vi "6-CleanFP.vi"   [LabVIEW 2014, in "TestVIs.lvlib"]
uses:
  TestVIs.lvlib
types:
  T1 = enum32{"Top Edges", "Vertical Centers", "Bottom Edges", "Vertical Gap", "Vertical Compress", "Left Edges", "Horizontal Centers", "Right Edges", "Horizontal Gap", "Horizontal Compress"}
  T2 = enum32{"Top Edges", "Vertical Centers", "Bottom Edges", "Left Edges", "Horizontal Centers", "Right Edges"}
  T3 = typedef "LVRectTypeDef.ctl" = cluster{"Left":i16, "Top":i16, "Right":i16, "Bottom":i16}
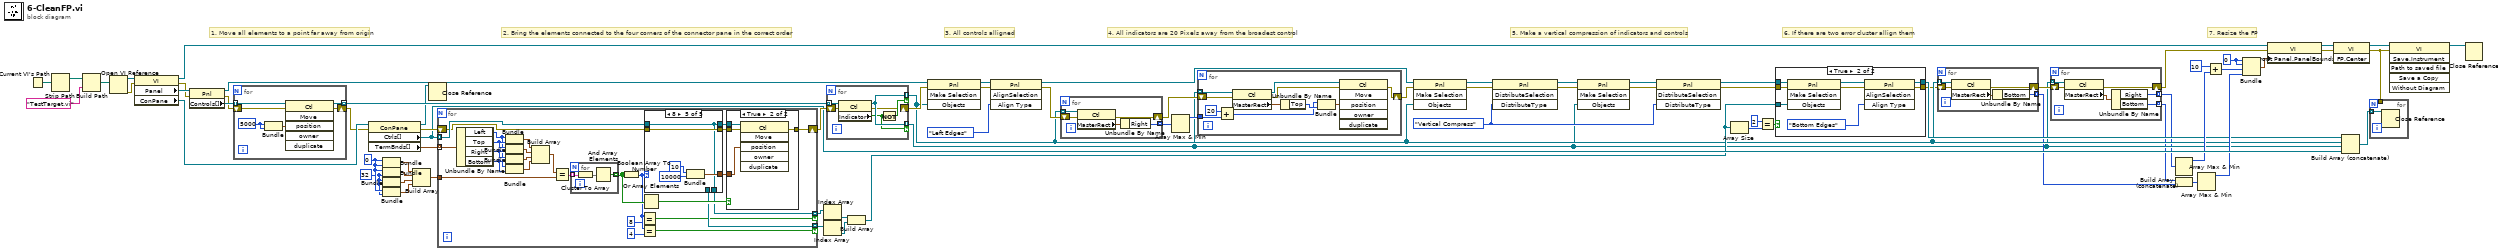
[diagram p0: block diagram]
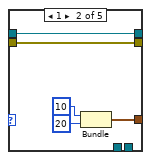
[diagram p4: hidden frame]
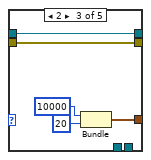
[diagram p5: hidden frame]
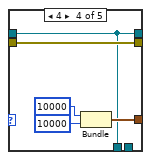
[diagram p6: hidden frame]
diagram:
  w19 = i16 0 ("x")
  w41 = i16 32
  w42 = i16 0
  w50 = T1."Vertical Compress" ("DistributeType")
  # "7. Resize the FP"
  # "6. If there are two error cluster allign them"
  # "2. Bring the elements connected to the four corners of the connector pane in the correct order"
  # "1. Move all elements to a point far away from origin"
  # "5. Make a vertical compression of indicators and controls"
  # "4. All indicators are 20 Pixels away from the broadest control"
  # "3. All controls alligned"
  n1 = Current VI's Path() -> (path=w72:path)
  n2 = Strip Path(path=w72) -> (stripped path=w75:path)  [unwired: 1 out]
  n3 = Build Path(base path=w75, name or relative path="TestTarget.vi") -> (appended path=w73:path)
  n4 = Open VI Reference(vi path=w73) -> (vi reference=w76:refnum<vi>, error out=w49:errorcluster)  [unwired: 5 in]
  n5 = property class="VI"(reference=w76, error in=w49) -> (reference out=w20:refnum<vi>, error out=w70:errorcluster, "Panel"=w71:refnum<vi>, "ConPane"=w45:refnum<vi>)
  n6 = property class="Pnl"(reference=w71, error in=w70) -> (reference out=w69:refnum<vi>, error out=w47:errorcluster, "Controls[]"=w48:refnum<vi>[])
  n7 = for {
    tunnel: w48 -> [w82] mode=indexing
    shift-right: [w80] -> w35
    shift-left: w47 -> [w81]
    tunnel: [w79] -> w46 mode=indexing
    w77 = i16 5000 ("x")
    n8 = Bundle("x"=w77, "x"=w77) -> (w78:cluster{"x":i16, "x":i16})  [unwired: 1 in]
    n9 = invoke class="Ctl" method="Move"(reference=w82, error in=w81, "position"=w78) -> (reference out=w79:refnum<vi>, error out=w80:errorcluster)  [unwired: 3 in, 4 out]
  }
  n10 = property class="ConPane"(reference=w45, error in=w35) -> (reference out=w34:refnum<vi>, error out=w43:errorcluster, "Ctrls[]"=w30:refnum<vi>[], "TermBnds[]"=w44:T3[])
  n11 = Bundle(w42, w42) -> (w40:cluster{i16, i16})  [unwired: 1 in]
  n12 = Bundle(w42, w41) -> (w39:cluster{i16, i16})  [unwired: 1 in]
  n13 = Bundle(w41, w41) -> (w38:cluster{i16, i16})  [unwired: 1 in]
  n14 = Bundle(w42, w41) -> (w37:cluster{i16, i16})  [unwired: 1 in]
  n15 = Build Array(w40, w39, w38, w37) -> (w36:cluster{i16, i16}[])
  n16 = Close Reference(reference=w34) -> ()  [unwired: 1 in, 1 out]
  n17 = for {
    tunnel: w44 -> [w109] mode=indexing
    tunnel: w30 -> [w92] mode=indexing
    tunnel: w36 -> [w99]
    shift-right: [w96] -> w33
    shift-left: w43 -> [w90]
    tunnel: [w89] -> w29 mode=indexing if=w84
    tunnel: [w88] -> w28 mode=indexing if=w83
    n18 = Unbundle By Name(w109) -> ("Left"=w106:i16, "Top"=w108:i16, "Right"=w107:i16, "Bottom"=w105:i16)
    n19 = Bundle("Left"=w106, "Top"=w108) -> (w101:cluster{"Left":i16, "Top":i16})  [unwired: 1 in]
    n20 = Bundle("Top"=w108, "Right"=w107) -> (w102:cluster{"Top":i16, "Right":i16})  [unwired: 1 in]
    n21 = Bundle("Right"=w107, "Bottom"=w105) -> (w103:cluster{"Right":i16, "Bottom":i16})  [unwired: 1 in]
    n22 = Bundle("Left"=w106, "Bottom"=w105) -> (w104:cluster{"Left":i16, "Bottom":i16})  [unwired: 1 in]
    n23 = Build Array(w101, w102, w103, w104) -> (w100:cluster{"Left":i16, "Bottom":i16}[])
    n24 = Equal?(x=w100, y=w99) -> (x = y?=w98:cluster{bool, bool}[])
    n25 = for {
      tunnel: w98 -> [w139] mode=indexing
      tunnel: [w137] -> w95 mode=indexing
      n26 = Cluster To Array(cluster=w139) -> (array=w138:bool[])
      n27 = And Array Elements(Boolean array=w138) -> (logical AND=w137:bool)
    }
    n28 = Boolean Array To Number(Boolean array=w95) -> (number=w87:u32)
    n29 = Equal?(x=w87, y=u32 8) -> (x = y?=w84:bool)
    n30 = Equal?(x=w87, y=u32 4) -> (x = y?=w83:bool)
    n31 = Or Array Elements(Boolean array=w95) -> (logical OR=w97:bool)
    n32 = case shown="8" w87 {
      tunnel: [_ w114 w119 w124 w129] -> w94
      tunnel: [w110 w113 w118 w122 w127] -> w93
      tunnel: w92 -> [w110 w113 w118 w122 w127]
      tunnel: [w111 w112 w117 w123 w128] -> w91
      tunnel: w90 -> [w111 w112 w117 w123 w128]
      tunnel: [_ _ _ _ w127] -> w89
      tunnel: [_ _ _ w122 _] -> w88
      frame 0, Default {
      }
      frame 1 {
        n33 = Bundle("x"=i16 10, "x"=i16 20) -> (w114:cluster{"x":i16, "x":i16})  [unwired: 1 in]
      }
      frame 2 {
        n34 = Bundle("x"=i16 10000, "x"=i16 20) -> (w119:cluster{"x":i16, "x":i16})  [unwired: 1 in]
      }
      frame 4 {
        n35 = Bundle("x"=i16 10000, "x"=i16 10000) -> (w124:cluster{"x":i16, "x":i16})  [unwired: 1 in]
      }
      frame 8 {
        n36 = Bundle("x"=i16 10, "x"=i16 10000) -> (w129:cluster{"x":i16, "x":i16})  [unwired: 1 in]
      }
    }
    n37 = case shown="True" w97 {
      tunnel: w93 -> [_ w136]
      tunnel: w91 -> [w132 w135]
      tunnel: [w132 w134] -> w96
      tunnel: w94 -> [_ w133]
      frame False {
      }
      frame True {
        n38 = invoke class="Ctl" method="Move"(reference=w136, error in=w135, "position"=w133) -> (error out=w134:errorcluster)  [unwired: 3 in, 5 out]
      }
    }
  }
  n39 = Index Array(array=w29) -> (element=w27:refnum<vi>)  [unwired: 1 in]
  n40 = Index Array(array=w28) -> (element=w26:refnum<vi>)  [unwired: 1 in]
  n41 = for {
    tunnel: w46 -> [w145] mode=indexing
    tunnel: [w144] -> w14 mode=indexing if=w143
    tunnel: [w144] -> w10 mode=indexing if=w142
    shift-right: [w140] -> w66
    shift-left: w33 -> [w141]
    n42 = property class="Ctl"(reference=w145, error in=w141) -> (reference out=w144:refnum<vi>, error out=w140:errorcluster, "Indicator"=w142:bool)
    n43 = Not(x=w142) -> (.not. x?=w143:bool)
  }
  n44 = Build Array(w27, w26) -> (w22:refnum<vi>[])
  n45 = invoke class="Pnl" method="Make Selection"(reference=w69, error in=w66, "Objects"=w14) -> (reference out=w68:refnum<vi>, error out=w67:errorcluster)  [unwired: 1 in, 2 out]
  n46 = invoke class="Pnl" method="AlignSelection"(reference=w68, error in=w67, "Align Type"=T2."Left Edges") -> (reference out=w57:refnum<vi>, error out=w59:errorcluster)  [unwired: 1 in, 2 out]
  n47 = for {
    tunnel: w14 -> [w150] mode=indexing
    tunnel: [w148] -> w62 mode=indexing
    shift-right: [w146] -> w60
    shift-left: w59 -> [w147]
    n48 = property class="Ctl"(reference=w150, error in=w147) -> (error out=w146:errorcluster, "MasterRect"=w149:T3)  [unwired: 1 out]
    n49 = Unbundle By Name(w149) -> ("Right"=w148:i16)
  }
  n50 = Array Max & Min(array=w62) -> (max value=w61:i16)  [unwired: 3 out]
  n51 = for {
    tunnel: w61 -> [w161]
    shift-right: [w153] -> w58
    shift-left: w60 -> [w158]
    tunnel: w10 -> [w159] mode=indexing
    n52 = Add(x=i16 20, y=w161) -> (x+y=w154:i16)
    n53 = property class="Ctl"(reference=w159, error in=w158) -> (reference out=w151:refnum<vi>, error out=w152:errorcluster, "MasterRect"=w157:T3)
    n54 = Unbundle By Name(w157) -> ("Top"=w155:i16)
    n55 = Bundle(w154, "Top"=w155) -> (w156:cluster{i16, "Top":i16})  [unwired: 1 in]
    n56 = invoke class="Ctl" method="Move"(reference=w151, error in=w152, "position"=w156) -> (error out=w153:errorcluster)  [unwired: 3 in, 5 out]
  }
  n57 = invoke class="Pnl" method="Make Selection"(reference=w57, error in=w58, "Objects"=w14) -> (reference out=w56:refnum<vi>, error out=w55:errorcluster)  [unwired: 1 in, 2 out]
  n58 = invoke class="Pnl" method="DistributeSelection"(reference=w56, error in=w55, "DistributeType"=w50) -> (reference out=w52:refnum<vi>, error out=w51:errorcluster)  [unwired: 1 in, 2 out]
  n59 = invoke class="Pnl" method="Make Selection"(reference=w52, error in=w51, "Objects"=w10) -> (reference out=w53:refnum<vi>, error out=w54:errorcluster)  [unwired: 1 in, 2 out]
  n60 = invoke class="Pnl" method="DistributeSelection"(reference=w53, error in=w54, "DistributeType"=w50) -> (reference out=w32:refnum<vi>, error out=w31:errorcluster)  [unwired: 1 in, 2 out]
  n61 = Array Size(array=w22) -> (size(s)=w25:i32)
  n62 = Equal?(x=2, y=w25) -> (x = y?=w23:bool)
  n63 = case shown="True" w23 {
    tunnel: w32 -> [w163 w171]
    tunnel: [w163 w170] -> w15
    tunnel: w31 -> [w162 w168]
    tunnel: [w162 w166] -> w13
    tunnel: w22 -> [_ w164]
    frame False {
    }
    frame True {
      n64 = invoke class="Pnl" method="Make Selection"(reference=w171, error in=w168, "Objects"=w164) -> (reference out=w169:refnum<vi>, error out=w167:errorcluster)  [unwired: 1 in, 2 out]
      n65 = invoke class="Pnl" method="AlignSelection"(reference=w169, error in=w167, "Align Type"=T2."Bottom Edges") -> (reference out=w170:refnum<vi>, error out=w166:errorcluster)  [unwired: 1 in, 2 out]
    }
  }
  n66 = for {
    tunnel: w14 -> [w176] mode=indexing
    shift-right: [w174] -> w11
    shift-left: w13 -> [w175]
    tunnel: [w172] -> w12 mode=indexing
    n67 = property class="Ctl"(reference=w176, error in=w175) -> (error out=w174:errorcluster, "MasterRect"=w173:T3)  [unwired: 1 out]
    n68 = Unbundle By Name(w173) -> ("Bottom"=w172:i16)
  }
  n69 = for {
    tunnel: w10 -> [w182] mode=indexing
    shift-right: [w180] -> w7
    shift-left: w11 -> [w181]
    tunnel: [w178] -> w9 mode=indexing
    tunnel: [w177] -> w8 mode=indexing
    n70 = property class="Ctl"(reference=w182, error in=w181) -> (error out=w180:errorcluster, "MasterRect"=w179:T3)  [unwired: 1 out]
    n71 = Unbundle By Name(w179) -> ("Right"=w178:i16, "Bottom"=w177:i16)
  }
  n72 = Array Max & Min(array=w9) -> (max value=w18:i16)  [unwired: 3 out]
  n73 = Build Array (concatenate)(w8, w12) -> (w21:i16[])
  n74 = Array Max & Min(array=w21) -> (max value=w17:i16)  [unwired: 3 out]
  n75 = Add(x=i16 10, y=w18) -> (x+y=w6:i16)
  n76 = Bundle("x"=w19, "x"=w19, w6, w17) -> (w16:cluster{"x":i16, "x":i16, i16, i16})  [unwired: 1 in]
  n77 = property class="VI"(reference=w20, error in=w7, "Front Panel.PanelBounds"=w16) -> (reference out=w4:refnum<vi>, error out=w2:errorcluster)
  n78 = invoke class="VI" method="FP.Center"(reference=w4, error in=w2) -> (reference out=w3:refnum<vi>, error out=w1:errorcluster)  [unwired: 1 in, 1 out]
  n79 = Build Array (concatenate)(w15, w14, w10, w30) -> (w63:refnum<vi>[])
  n80 = for {
    tunnel: w1 -> [_]
    tunnel: w63 -> [w183] mode=indexing
    n81 = Close Reference(reference=w183) -> ()  [unwired: 1 in, 1 out]
  }
  n82 = invoke class="VI" method="Save.Instrument"(reference=w3, error in=w1) -> (reference out=w64:refnum<vi>)  [unwired: 4 in, 5 out]
  n83 = Close Reference(reference=w64) -> ()  [unwired: 1 in, 1 out]
